vi "VPA QC Add Comment.vi"(8 "error in (no error)":errorcluster, 10 "State Cluster In":T1) -> (0 "error out":errorcluster, 2 "State Cluster Out":T1)   [LabVIEW 2013]
uses:
  Controls/VPA QC State Data Cluster.ctl
  Controls/VPA QC General Cluster.ctl
  Controls/VPA QC State Enum.ctl
  Controls/VPA QC Bool Cluster.ctl
panel:
  in  "Cancel":bool
  in  "Save":bool
  in  "Comment":string
  in  "Time and Date":timestamp
  # "Assembly Checklist"
  # "Assembly Checklist"
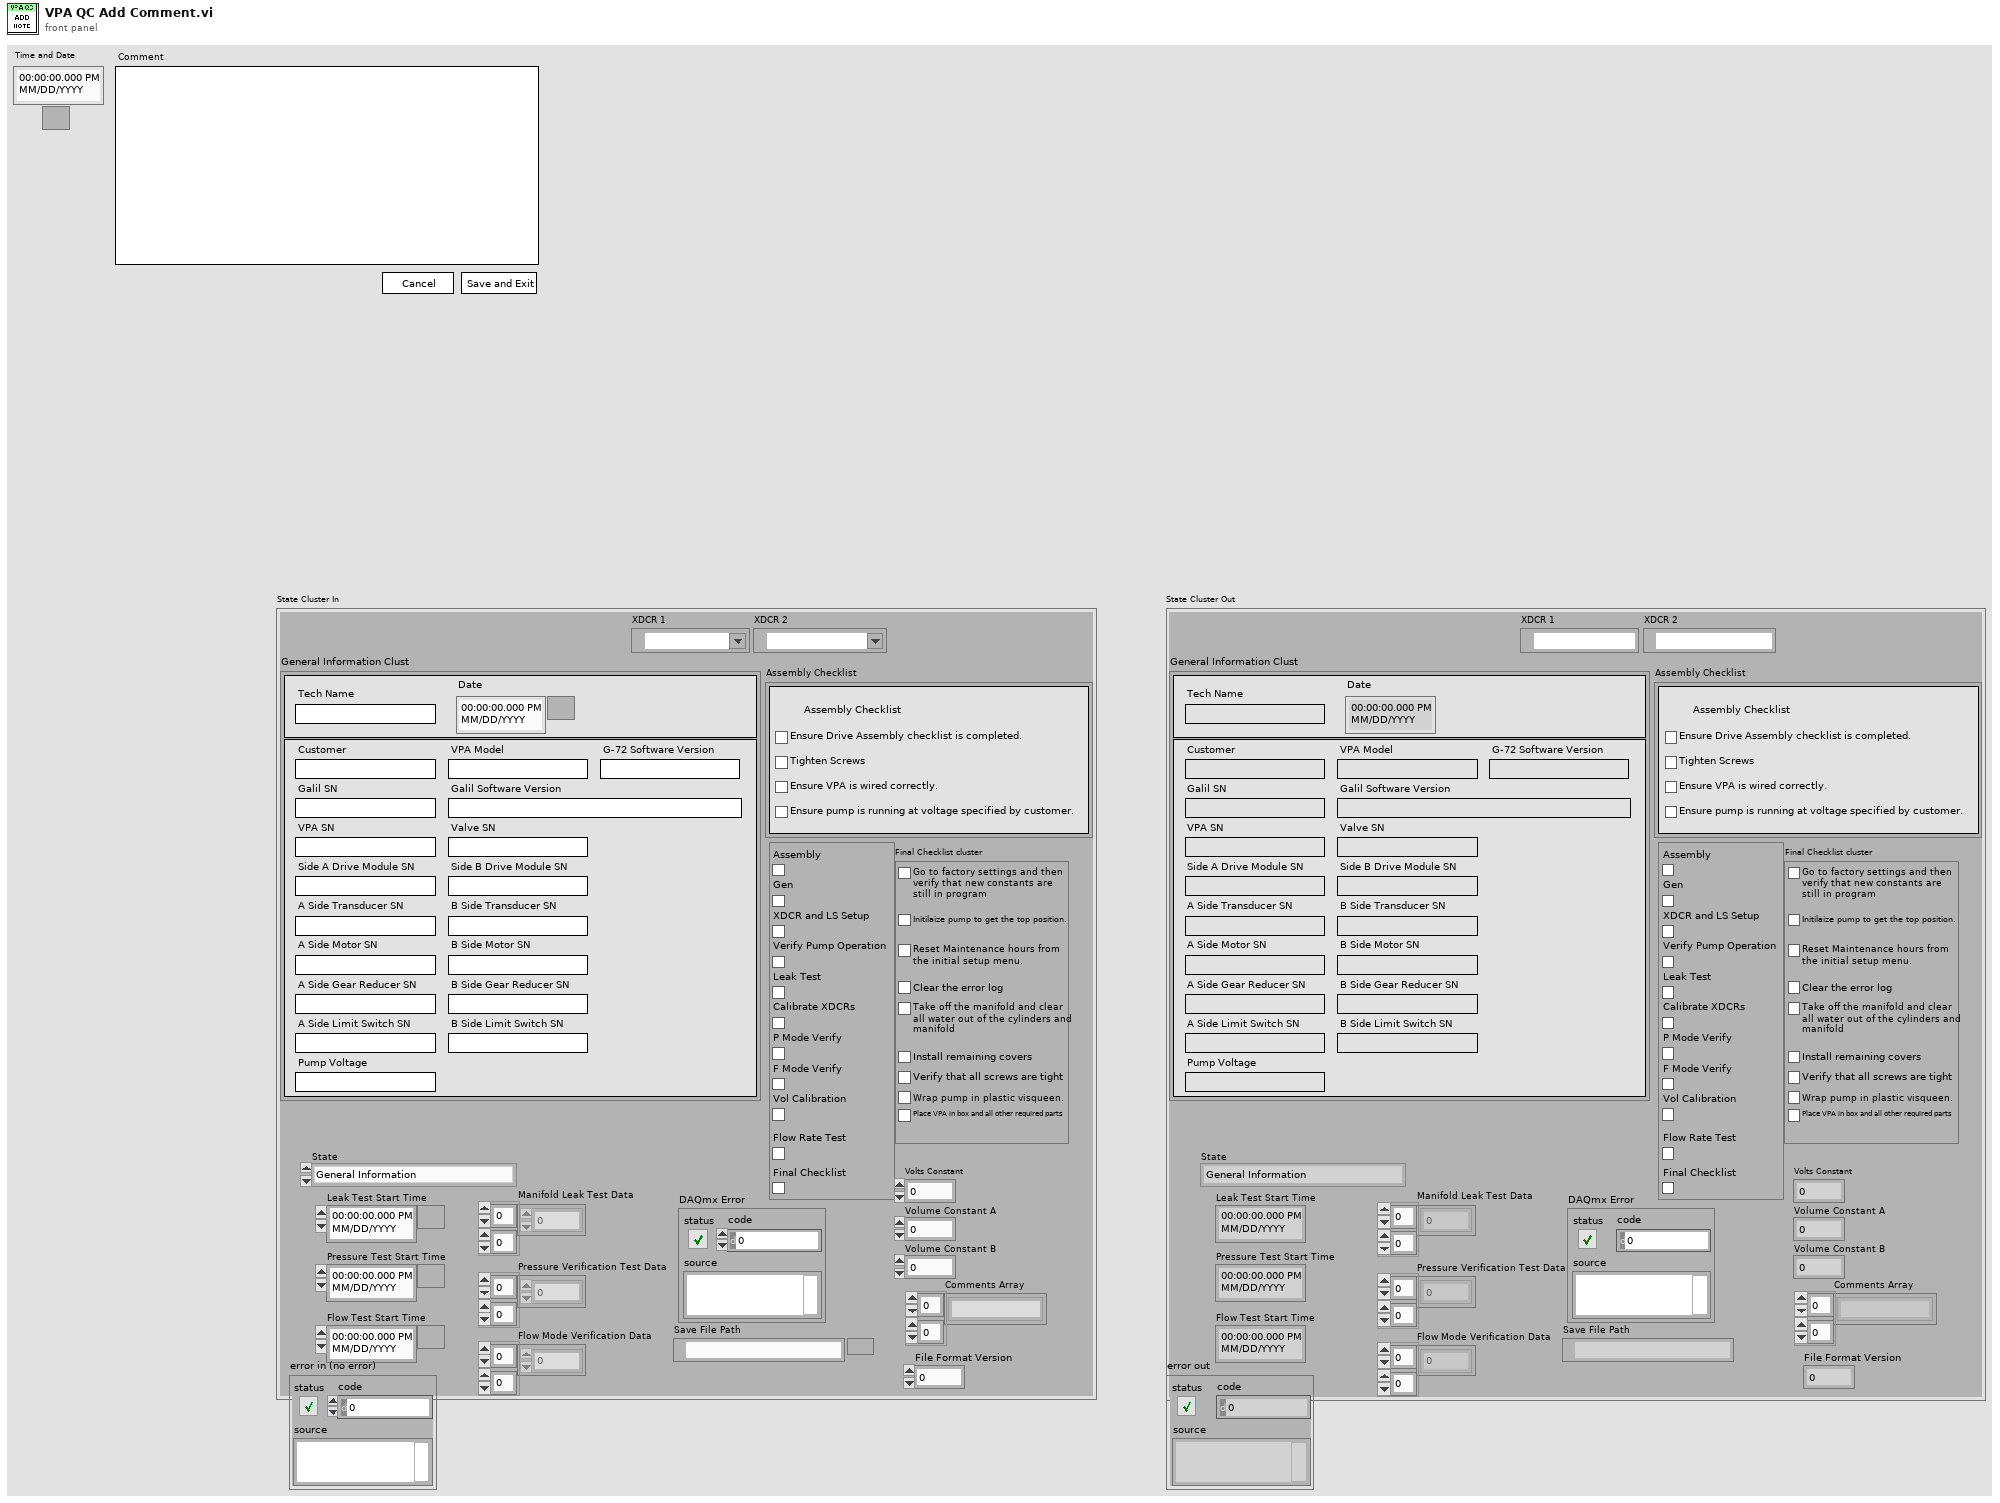
[diagram p1: front panel]
types:
  T1 = typedef "VPA QC State Data Cluster.ctl" = cluster{"XDCR 1":tag, "XDCR 2":tag, "General Information Clust":T2, "Assembly Checklist":cluster{"Ensure Drive Assembly checklist is completed.":bool, "Tighten Screws":bool, "Ensure VPA is wired correctly.":bool, "Ensure pump is running at voltage specified by customer.":bool}, "State":T3, "Manifold Leak Test Data":dbl[][], "Pressure Verification Test Data":dbl[][], "Flow Mode Verification Data":dbl[][], "DAQmx Error":errorcluster, "Bool Cluster":T4, "Leak Test Start Time":timestamp, "Pressure Test Start Time":timestamp, "Flow Test Start Time":timestamp, "Final Checklist cluster":cluster{"Check Fact Rest":bool, "Initialize Pump":bool, "Maintenance Hours":bool, "Clean Water Out":bool, "Covers":bool, "Screws":bool, "Wrap":bool, "Box":bool, "Clear Error Log":bool}, "Volts Constant":dbl, "Volume Constant A":dbl, "Volume Constant B":dbl, "Save File Path":path, "Comments Array":string[][], "File Format Version":u16}
  T2 = typedef "VPA QC General Cluster.ctl" = cluster{"Tech Name":string, "Date":timestamp, "Customer":string, "VPA Model":string, "G-72 Software Version":string, "Galil SN":string, "Galil Software Version":string, "VPA SN":string, "Valve SN":string, "Side A Drive Module SN":string, "Side B Drive Module SN":string, "A Side Transducer SN":string, "B Side Transducer SN":string, "A Side Motor SN":string, "B Side Motor SN":string, "A Side Gear Reducer SN":string, "B Side Gear Reducer SN":string, "A Side Limit Switch SN":string, "B Side Limit Switch SN":string, "Pump Voltage":string}
  T3 = typedef "VPA QC State Enum.ctl" = enum16{"General Information", "XDCR and LS Check", "Check Pump Function", "Manifold/Cylinder Leak Test", "Exit"}
  T4 = typedef "VPA QC Bool Cluster.ctl" = cluster{"Assembly":bool, "Gen":bool, "XDCR and LS Setup":bool, "Verify Pump Operation":bool, "Leak Test":bool, "Calibrate XDCRs":bool, "P Mode Verify":bool, "F Mode Verify":bool, "Vol Calibration":bool, "Flow Rate Test":bool, "Final Checklist":bool}
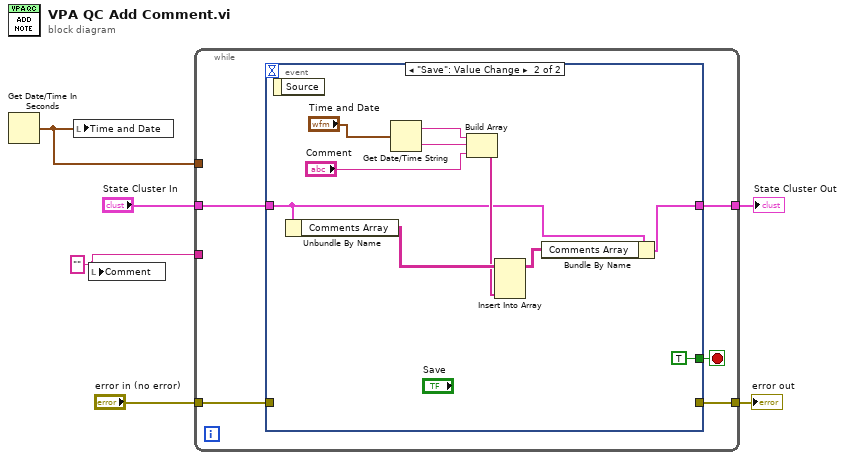
[diagram p0: block diagram]
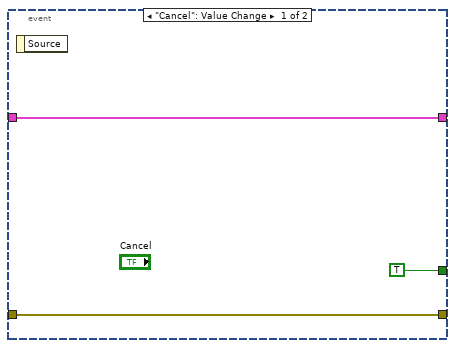
[diagram p2: hidden frame]
diagram:
  w1 = "" ("Comment")
  n1 = Get Date/Time In Seconds() -> (seconds since 1Jan1904=w2:timestamp)
  n2 = local write "Time and Date"(w2) -> ()
  n3 = local write "Comment"(w1) -> ()
  n4 = while {
    tunnel: "State Cluster In" -> [w11]
    tunnel: [w10] -> w3
    tunnel: "error in (no error)" -> [w8]
    tunnel: [w7] -> w4
    tunnel: w2 -> [_]
    tunnel: w1 -> [_]
    stop <- w9 stop-if-true
    n5 = event shown="[1] \"Save\": Value Change" {
      selector: _ -> [_ _]
      dyn-events: _ -> [_ _]
      timeout: _ -> [_ _]
      tunnel: w11 -> [w14 w18]
      tunnel: [w14 w17] -> w10
      tunnel: [TRUE TRUE] -> w9
      tunnel: [w12 _] -> w7
      tunnel: w8 -> [w12 _]
      event "Cancel": Value Change {
        n6 = event-data() -> ()  [unwired: 1 in, 1 out]
      }
      event "Save": Value Change {
        n7 = event-data() -> ()  [unwired: 1 in, 1 out]
        n8 = Unbundle By Name(w18) -> ("Comments Array"=w23:string[][])
        n9 = Get Date/Time String(seconds (now)="Time and Date") -> (date string=w22:string, time string=w21:string)  [unwired: 2 in]
        n10 = Build Array(w22, w21, "Comment") -> (w19:string[])
        n11 = Insert Into Array(array=w23, new element=w19) -> (w16:string[][])  [unwired: 2 in]
        n12 = Bundle By Name(cluster=w18, "Comments Array"=w16) -> (w17:T1)
      }
    }
  }
  "State Cluster Out" <- w3
  "error out" <- w4
